vi "PopupWindowHandler.vi"(10 "AscriptRefs":T1, 11 "BasePath":path) -> ()   [LabVIEW 2015]
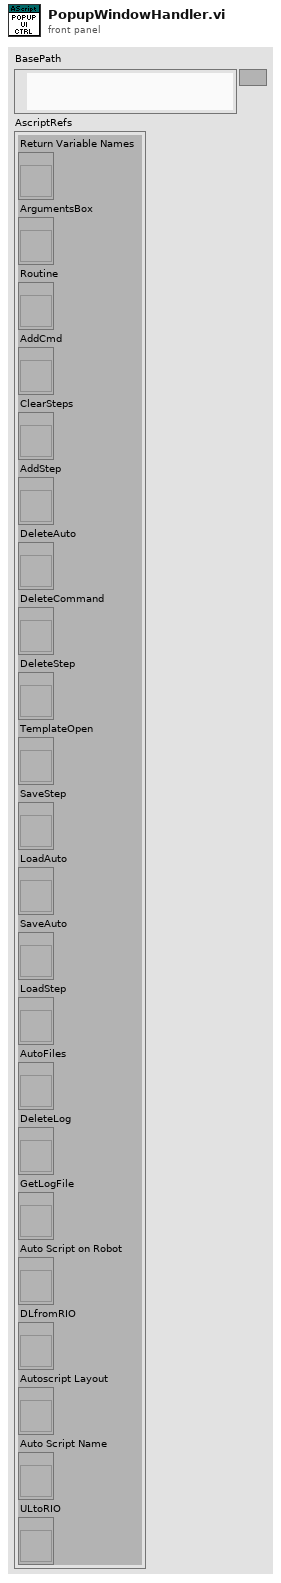
[diagram p1: front panel]
types:
  T1 = cluster{"Return Variable Names":refnum<vi>, "ArgumentsBox":refnum<vi>, "Routine":refnum<vi>, "AddCmd":refnum<vi>, "ClearSteps":refnum<vi>, "AddStep":refnum<vi>, "DeleteAuto":refnum<vi>, "DeleteCommand":refnum<vi>, "DeleteStep":refnum<vi>, "TemplateOpen":refnum<vi>, "SaveStep":refnum<vi>, "LoadAuto":refnum<vi>, "SaveAuto":refnum<vi>, "LoadStep":refnum<vi>, "AutoFiles":refnum<vi>, "DeleteLog":refnum<vi>, "GetLogFile":refnum<vi>, "Auto Script on Robot":refnum<vi>, "DLfromRIO":refnum<vi>, "Autoscript Layout":refnum<vi>, "Auto Script Name":refnum<vi>, "ULtoRIO":refnum<vi>}
  T2 = cluster{"Number":i32, "Name":string, "Commands":string[], "WaitForExecution":bool}
  T3 = cluster{"Number":i32, "Name":string, "Commands":string[], "WaitForExecution":bool}[]
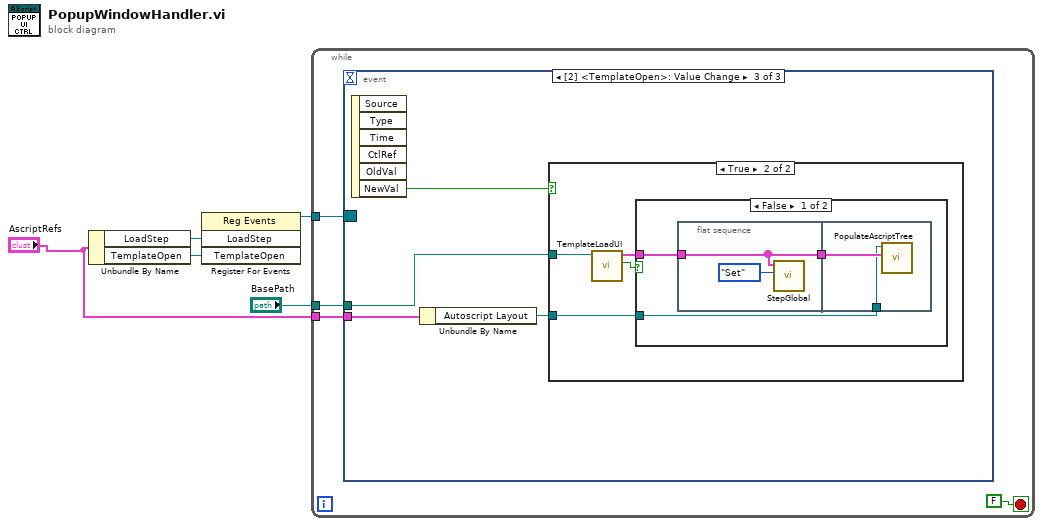
[diagram p0: block diagram]
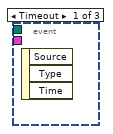
[diagram p2: hidden frame]
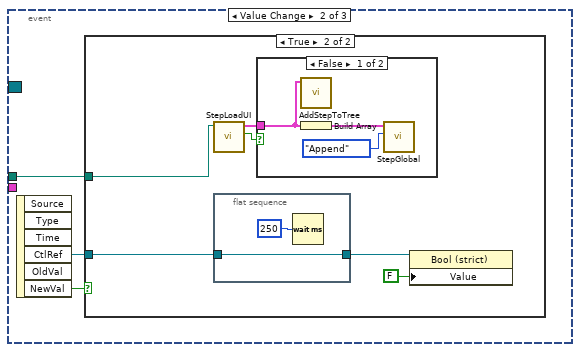
[diagram p3: hidden frame]
diagram:
  n1 = Unbundle By Name("AscriptRefs") -> ("LoadStep"=w4:refnum<vi>, "TemplateOpen"=w3:refnum<vi>)
  n2 = register-events(w4, w3) -> (reference out=w5:refnum<event-registration>)  [unwired: 2 in, 1 out]
  n3 = while {
    tunnel: w5 -> [w9]
    tunnel: "AscriptRefs" -> [w7]
    tunnel: "BasePath" -> [w6]
    stop <- FALSE stop-if-true
    n4 = event shown="[2] <TemplateOpen>: Value Change" {
      selector: w9 -> [_ _ _]
      dyn-events: _ -> [_ _ _]
      timeout: _ -> [_ _ _]
      tunnel: w7 -> [_ _ w27]
      tunnel: w6 -> [_ w10 w24]
      event Timeout {
        n5 = event-data() -> ()  [unwired: 1 in, 3 out]
      }
      event Value Change {
        n6 = event-data() -> ("CtlRef"=w11:refnum<vi>, "NewVal"=w12:bool)  [unwired: 1 in, 4 out]
        n7 = case shown="True" w12 {
          tunnel: w11 -> [_ w18]
          tunnel: w10 -> [_ w13]
          frame False {
          }
          frame True {
            n8 = call "StepLoadUI.vi"("base path"=w13) -> ("Cancelled?"=w14:bool, "Step"=w15:T2)  [unwired: 9 in]
            n9 = flat-sequence {
              tunnel: w18 -> [w22]
              tunnel: [w22] -> w17
              frame #0 {
                n10 = Wait (ms)(milliseconds to wait=u32 250) -> ()  [unwired: 1 out]
              }
            }
            n11 = case shown="False" w14 {
              tunnel: w15 -> [w20 _]
              frame False {
                n12 = call "AddStepToTree.vi"("Step"=w20) -> ()  [unwired: 10 in, 1 out]
                n13 = Build Array(w20) -> (w19:T3)
                n14 = call "StepGlobal.vi"("Action (Get)"=enum16{"Clear", "Append", "Set", "Get"}."Append" ("Action"), "AutoScriptSteps in"=w19) -> ()  [unwired: 9 in, 1 out]
              }
              frame True {
              }
            }
            n15 = property class="Bool (strict)"(reference=w17, "Value"=FALSE) -> ()  [unwired: 1 in, 2 out]
          }
        }
      }
      event Value Change {
        n16 = event-data() -> ("NewVal"=w25:bool)  [unwired: 1 in, 5 out]
        n17 = Unbundle By Name(w27) -> ("Autoscript Layout"=w26:refnum<vi>)
        n18 = case shown="True" w25 {
          tunnel: w26 -> [_ w29]
          tunnel: w24 -> [_ w28]
          frame False {
          }
          frame True {
            n19 = call "TemplateLoadUI.vi"("BasePath"=w28) -> ("Cancelled?"=w31:bool, "Steps"=w30:T3)  [unwired: 9 in]
            n20 = case shown="False" w31 {
              tunnel: w30 -> [w34 _]
              tunnel: w29 -> [w32 _]
              frame False {
                n21 = flat-sequence {
                  tunnel: w34 -> [w35]
                  tunnel: [w35] -> w33
                  tunnel: w33 -> [w38]
                  tunnel: w32 -> [w37]
                  frame #0 {
                    n22 = call "StepGlobal.vi"("Action (Get)"=enum16{"Clear", "Append", "Set", "Get"}."Set" ("Action"), "AutoScriptSteps in"=w35) -> ()  [unwired: 9 in, 1 out]
                  }
                  frame #1 {
                    n23 = call "PopulateAscriptTree.vi"("Steps in"=w38, "Autoscript Layout"=w37) -> ()  [unwired: 8 in, 2 out]
                  }
                }
              }
              frame True {
              }
            }
          }
        }
      }
    }
  }
